vi "CP_Find_Child_Ref_from_Array.vi"(0 "Child_Ref Array":T1[](array[typedef]), 7 "Queue ID":string, 11 "error in (no error)":errorcluster) -> (3 "Found?":bool, 4 "Child_Ref out":refnum<vi>, 6 "SubPanel Ref":refnum<vi>, 8 "Child Queue":refnum<queue>, 10 "Parent Queue":refnum<queue>, 15 "error out":errorcluster)   [LabVIEW 2009]
doc: "Part of the Dock/Undock demonstration of Sub Panels. Contributed by www.entzen.com.\n\nAAL 9/09"
uses:
  TD_Child_Ref_Cluster.ctl
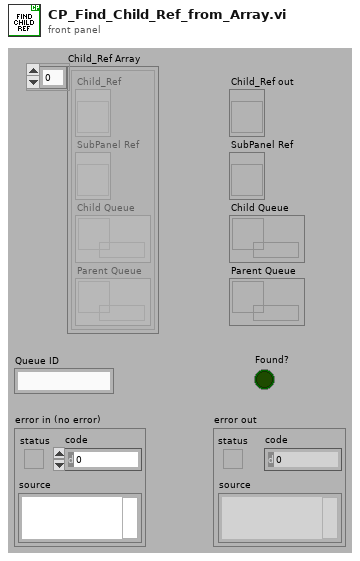
[diagram p1: front panel]
types:
  T1 = typedef "TD_Child_Ref_Cluster.ctl" = cluster{"Child_Ref":refnum<vi>, "SubPanel Ref":refnum<vi>, "Child Queue":refnum<queue>, "Parent Queue":refnum<queue>}
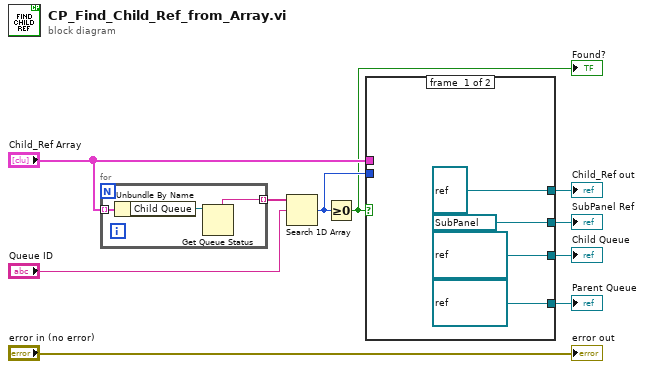
[diagram p0: block diagram]
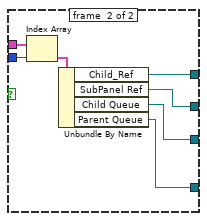
[diagram p2: hidden frame]
diagram:
  n1 = for {
    tunnel: "Child_Ref Array" -> [w13] mode=indexing
    tunnel: [w11] -> w10 mode=indexing
    n2 = Unbundle By Name(w13) -> ("Child Queue"=w12:refnum<queue>)
    n3 = Get Queue Status(queue=w12) -> (queue name=w11:string)  [unwired: 2 in, 7 out]
  }
  n4 = Search 1D Array(1D array=w10, element="Queue ID") -> (index of element=w6:i32)  [unwired: 1 in]
  n5 = Greater Or Equal To 0?(x=w6) -> (x >= 0?=w5:bool)
  "Found?" <- w5
  n6 = case shown="True" w5 {
    tunnel: "Child_Ref Array" -> [_ w24]
    tunnel: w6 -> [_ w23]
    tunnel: [refnum<vi> refnum ("Child_Ref") w21] -> w4
    tunnel: [refnum<queue> refnum ("Child Queue") w20] -> w3
    tunnel: [refnum<queue> refnum ("Child Queue") w19] -> w2
    tunnel: [refnum<vi> refnum ("SubPanel Ref") w18] -> w1
    frame #0 {
    }
    frame #1 {
      n7 = Index Array(array=w24, index=w23) -> (element=w22:T1)
      n8 = Unbundle By Name(w22) -> ("Child_Ref"=w21:refnum<vi>, "SubPanel Ref"=w18:refnum<vi>, "Child Queue"=w20:refnum<queue>, "Parent Queue"=w19:refnum<queue>)
    }
  }
  "Child_Ref out" <- w4
  "Child Queue" <- w3
  "Parent Queue" <- w2
  "SubPanel Ref" <- w1
  "error out" <- "error in (no error)"
